vi "Log Data.vi"(6 "Samples to Save In":u32, 7 "Logging Configuration":T3, 8 "error in (no error)":errorcluster, 9 "Data":waveform(dbl)[](array[waveform]), 10 "Piezo Data":T2, 11 "Cap Data":T1) -> (0 "error out":errorcluster, 4 "Samples to Save Out":u32)   [LabVIEW 2013, in "Logging.lvlib"]
doc: "Use the Write To Measurement File Express VI to log data to disk in a LVM file."
uses:
  Logging.lvlib
  Logging Configuration.ctl
  Piezo/Piezo display.ctl
  Capacitive/Capacitive Signal Cluster.ctl
  Piezo/Piezo.lvlib
  Capacitive/Capacitive.lvlib
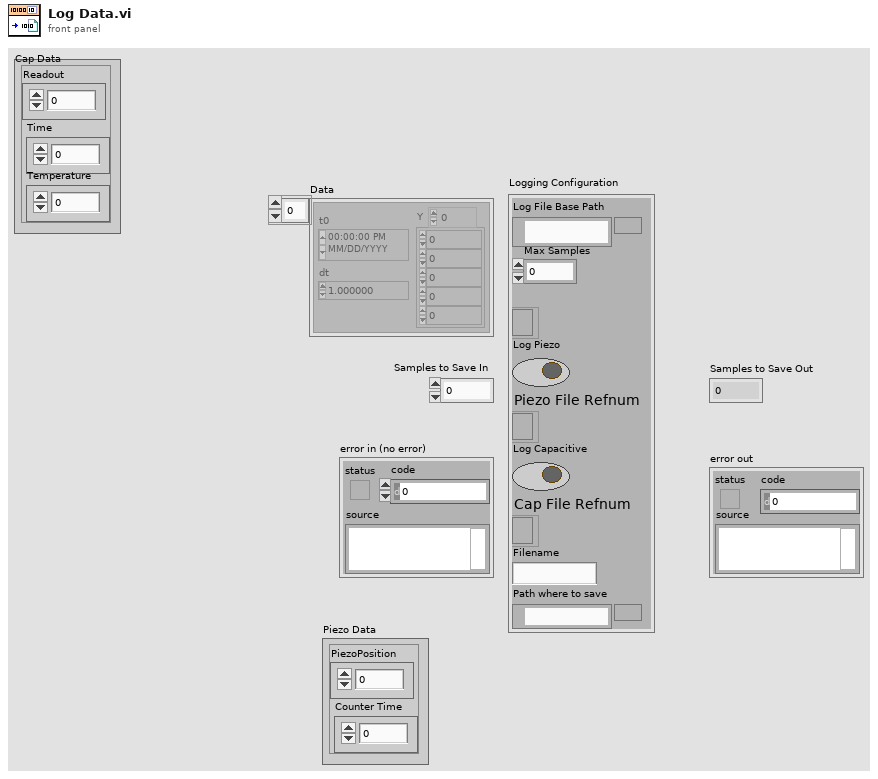
[diagram p1: front panel]
types:
  T1 = typedef "Capacitive.lvlib/Capacitive Signal Cluster.ctl" = cluster{"Readout":sgl, "Time":i32, "Temperature":dbl}
  T2 = typedef "Piezo.lvlib/Piezo display.ctl" = cluster{"PiezoPosition":sgl, "Counter Time":i32}
  T3 = typedef "Logging.lvlib/Logging Configuration.ctl" = cluster{"Log File Base Path":path, "Max Samples":u32, "File Refnum":refnum<file>, "Log Piezo":bool, "Piezo File Refnum":refnum<file>, "Log Capacitive":bool, "Cap File Refnum":refnum<file>, "Filename":string, "Path where to save":path}
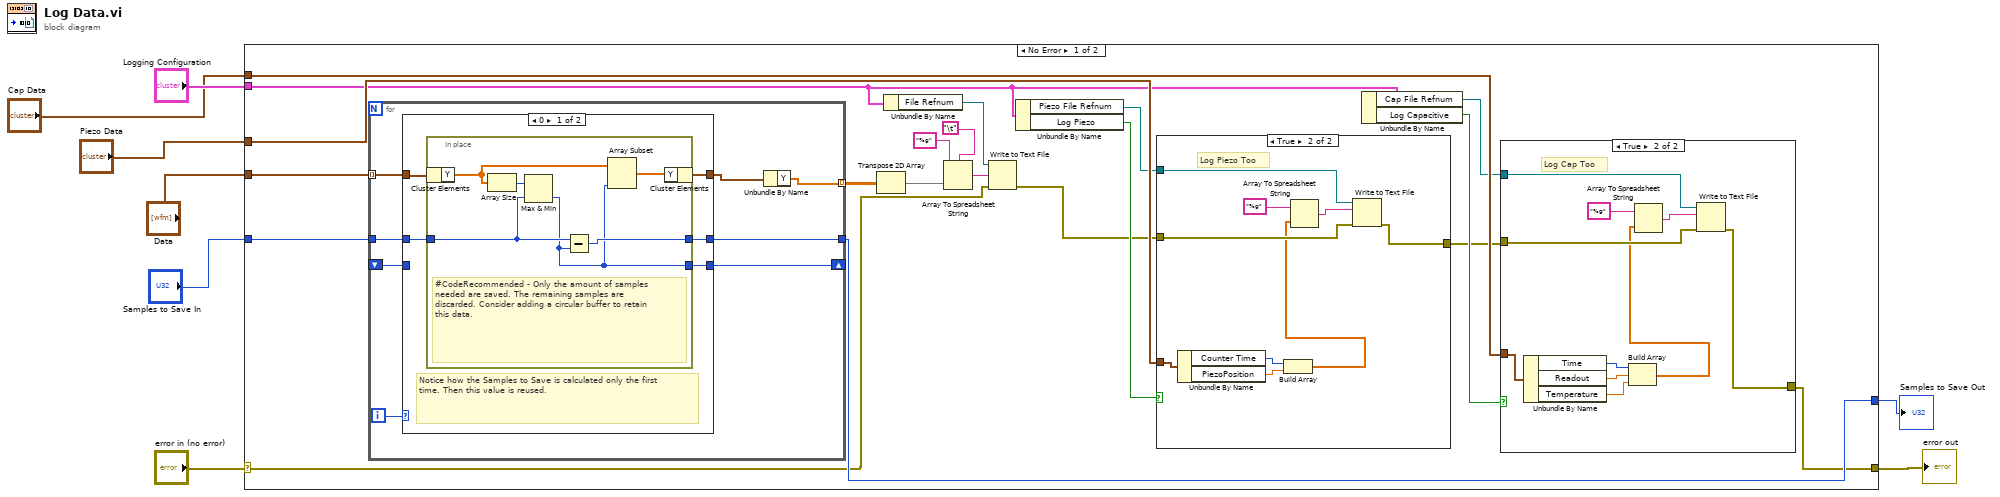
[diagram p0: block diagram]
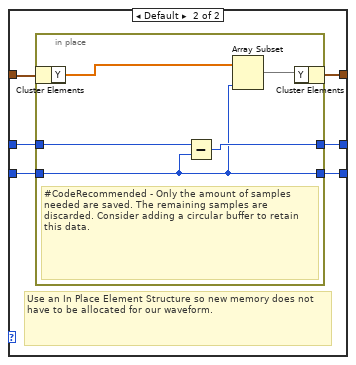
[diagram p4: hidden frame]
diagram:
  n1 = case shown="No Error" "error in (no error)" {
    selector: "error in (no error)" -> [w18 w81]
    tunnel: "Logging Configuration" -> [w14 _]
    tunnel: "Data" -> [w28 _]
    tunnel: [w9 w81] -> w7
    tunnel: "Samples to Save In" -> [w27 w80]
    tunnel: [w26 w80] -> w3
    tunnel: "Piezo Data" -> [w21 _]
    tunnel: "Cap Data" -> [w13 _]
    frame No Error {
      n2 = for {
        tunnel: w28 -> [w56] mode=indexing
        tunnel: w27 -> [w57]
        tunnel: [w55] -> w26
        shift-right: [w53] -> _
        shift-left: _ -> [w52]
        tunnel: [w50] -> w17 mode=indexing
        i -> [w54]
        n3 = case shown="0" w54 {
          tunnel: w57 -> [w62 w74]
          tunnel: w56 -> [w58 w70]
          tunnel: [w59 w69] -> w51
          tunnel: [w61 w73] -> w55
          tunnel: [w60 w71] -> w53
          tunnel: w52 -> [_ w72]
          frame 0 {
            # "Notice how the Samples to Save is calculated only the first time. Then this value is reused."
            n4 = in-place {
              in-place-border: w62 -> [w67]
              in-place-border: [w66] -> w61
              in-place-border: [w63] -> w60
              # "#CodeRecommended - Only the amount of samples needed are saved. The remaining samples are discarded. Consider adding a circular buffer to retain this data."
              n5 = in-place-cluster #1(w58) -> ("Y"=w65:dbl[])
              n6 = Array Size(array=w65) -> (size(s)=w68:i32)
              n7 = Max & Min(x=w68, y=w67) -> (min(x,y)=w63:u32)  [unwired: 1 out]
              n8 = Subtract(x=w67, y=w63) -> (x-y=w66:u32)
              n9 = Array Subset(array=w65, length=w63) -> (w64:dbl[])  [unwired: 1 in]
              n10 = in-place-cluster #1("Y"=w64) -> (w59:waveform(dbl))
            }
          }
          frame Default {
            # "Use an In Place Element Structure so new memory does not have to be allocated for our waveform."
            n11 = in-place {
              in-place-border: w74 -> [w79]
              in-place-border: [w78] -> w73
              in-place-border: [w75] -> w71
              in-place-border: w72 -> [w75]
              # "#CodeRecommended - Only the amount of samples needed are saved. The remaining samples are discarded. Consider adding a circular buffer to retain this data."
              n12 = in-place-cluster #2(w70) -> ("Y"=w77:dbl[])
              n13 = Subtract(x=w79, y=w75) -> (x-y=w78:u32)
              n14 = Array Subset(array=w77, length=w75) -> (w76:dbl[])  [unwired: 1 in]
              n15 = in-place-cluster #2("Y"=w76) -> (w69:waveform(dbl))
            }
          }
        }
        n16 = Unbundle By Name(w51) -> ("Y"=w50:dbl[])
      }
      n17 = Transpose 2D Array(2D array=w17) -> (transposed array=w16:dbl[][])
      n18 = Unbundle By Name(w14) -> ("File Refnum"=w25:refnum<file>)
      n19 = Array To Spreadsheet String(delimiter (Tab)="\t", array=w16, 3:"%g" ("format string")) -> (spreadsheet string=w24:string)
      n20 = Write to Text File(file (use dialog)=w25, text=w24, error in=w18) -> (error out=w19:errorcluster)  [unwired: 1 in, 2 out]
      n21 = Unbundle By Name(w14) -> ("Piezo File Refnum"=w20:refnum<file>, "Log Piezo"=w22:bool)
      n22 = case shown="True" w22 {
        tunnel: w21 -> [_ w47]
        tunnel: w20 -> [_ w49]
        tunnel: w19 -> [w40 w43]
        tunnel: [w40 w42] -> w10
        frame False {
        }
        frame True {
          # "Log Piezo Too"
          n23 = Unbundle By Name(w47) -> ("Counter Time"=w46:i32, "PiezoPosition"=w45:sgl)
          n24 = Build Array(w46, w45) -> (w41:sgl[])
          n25 = Array To Spreadsheet String(array=w41, 3:"%g" ("format string")) -> (spreadsheet string=w48:string)  [unwired: 1 in]
          n26 = Write to Text File(file (use dialog)=w49, text=w48, error in=w43) -> (error out=w42:errorcluster)  [unwired: 1 in, 2 out]
        }
      }
      n27 = Unbundle By Name(w14) -> ("Cap File Refnum"=w12:refnum<file>, "Log Capacitive"=w11:bool)
      n28 = case shown="True" w11 {
        tunnel: w12 -> [_ w39]
        tunnel: w10 -> [w29 w34]
        tunnel: [w29 w33] -> w9
        tunnel: w13 -> [_ w31]
        frame False {
        }
        frame True {
          # "Log Cap Too"
          n29 = Unbundle By Name(w31) -> ("Time"=w37:i32, "Readout"=w36:sgl, "Temperature"=w30:dbl)
          n30 = Build Array(w37, w36, w30) -> (w32:dbl[])
          n31 = Array To Spreadsheet String(array=w32, 3:"%g" ("format string")) -> (spreadsheet string=w38:string)  [unwired: 1 in]
          n32 = Write to Text File(file (use dialog)=w39, text=w38, error in=w34) -> (error out=w33:errorcluster)  [unwired: 1 in, 2 out]
        }
      }
    }
    frame Error {
    }
  }
  "error out" <- w7
  "Samples to Save Out" <- w3
